vi "Create Waveforms.vi"(0 "RFFE Command in":refnum<class "RFFE Command.lvclass">, 5 "instrument handle in":refnum<k15>, 11 "error in (no error)":errorcluster) -> (4 "RFFE Command out":refnum<class "RFFE Command.lvclass">, 6 "instrument handle out":refnum<k15>, 15 "error out":errorcluster)   [LabVIEW 2018, in "MIPI RFFE API.lvlib" / "RFFE Command.lvclass"]
uses:
  RFFE Command.lvclass
  <instrlib>/niDigital/niDigital.llb/niDigital Data Mapping.ctl
  RFFE Command.lvclass/RFFE Command.ctl
  <instrlib>/niDigital/niDigital.llb/niDigital Create Source Waveform (Serial).vi
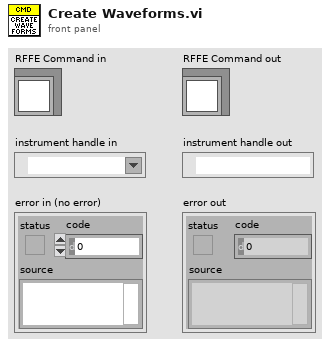
[diagram p1: front panel]
types:
  T1 = typedef "niDigital Data Mapping.ctl" = i32
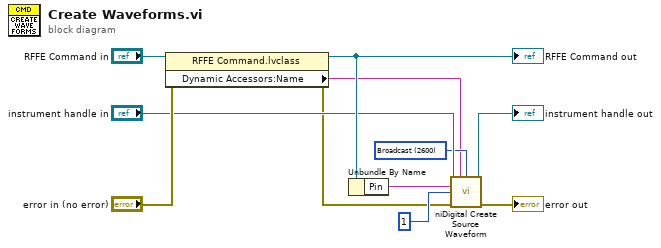
[diagram p0: block diagram]
diagram:
  w5 = T1 2600 items=["Broadcast"=2600, "Site Unique"=2601] ("data mapping")
  n1 = property class="RFFE Command.lvclass"(reference="RFFE Command in", error in="error in (no error)") -> (reference out=w8:refnum<class "RFFE Command.lvclass">, error out=w1:errorcluster, "Dynamic Accessors:Name"=w2:string)
  "RFFE Command out" <- w8
  n2 = Unbundle By Name(w8) -> ("Pin"=w3:string)
  n3 = call-poly <instrlib>:"niDigital Create Source Waveform.vi"("instrument handle"="instrument handle in", "waveform name"=w2, "data mapping"=w5, "pin list"=w3, "sample width"=u32 1, "error in"=w1) -> ("instrument handle out"=→"instrument handle out":refnum<k15>, "error out"=→"error out":errorcluster)  [unwired: 8 in]
